vi "New Analog Edge Trigger.vi"(7 "Slope":T1, 8 "error in (no error)":errorcluster, 10 "Strict Edge":bool, 11 "Threshold":dbl) -> (0 "error out":errorcluster, 3 "Analog Edge Trigger out":refnum<class "Analog Edge Trigger.lvclass">)   [LabVIEW 2015, in "Waveform Data Logger Engine.lvlib" / "Analog Edge Trigger.lvclass"]
uses:
  Analog Edge Trigger.lvclass
  Analog Slope Type.ctl
  Analog Edge Trigger.lvclass/Analog Edge Trigger.ctl
  Trigger/Trigger Type.ctl
  Trigger/Trigger.lvclass/Trigger.ctl
  Trigger/Write Trigger Type.vi
  Trigger/Trigger.lvclass
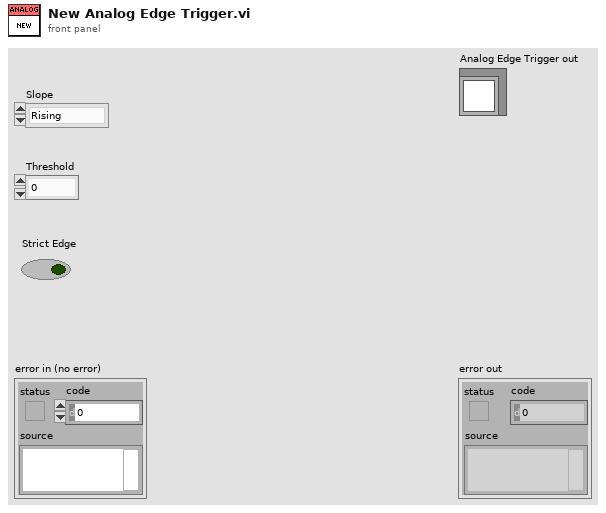
[diagram p1: front panel]
types:
  T1 = typedef "Waveform Data Logger Engine.lvlib/Analog Edge Trigger.lvclass/Analog Slope Type.ctl" = enum16{"Rising", "Falling"}
  T2 = typedef "Waveform Data Logger Engine.lvlib/Trigger.lvclass/Trigger Type.ctl" = enum16{"Default", "Digital Edge", "Analog Edge", "In Range", "Value Change", "Boolean Evaluation"}
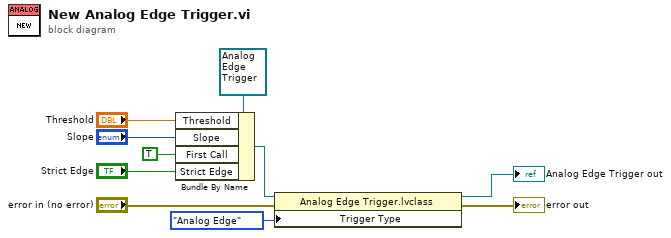
[diagram p0: block diagram]
diagram:
  n1 = Bundle By Name(cluster=refnum<class "Analog Edge Trigger.lvclass"> refnum ("Analog Edge Trigger in"), "Threshold"="Threshold", "Slope"="Slope", "First Call"=TRUE, "Strict Edge"="Strict Edge") -> (w5:refnum<class "Analog Edge Trigger.lvclass">)
  n2 = property class="Analog Edge Trigger.lvclass"(reference=w5, error in="error in (no error)", "Trigger Type"=Trigger_Type."Analog Edge") -> (reference out=→"Analog Edge Trigger out":refnum<class "Analog Edge Trigger.lvclass">, error out=→"error out":errorcluster)
